vi "chart_combined.vi"() -> ()   [LabVIEW 8.6]
uses:
  Controls/lxw_chart_type.ctl
  Controls/lxw_chart_axis_type.ctl
panel:
  out "error out":errorcluster
  out "function return 2":string
  # "chart_combined.xlsx"
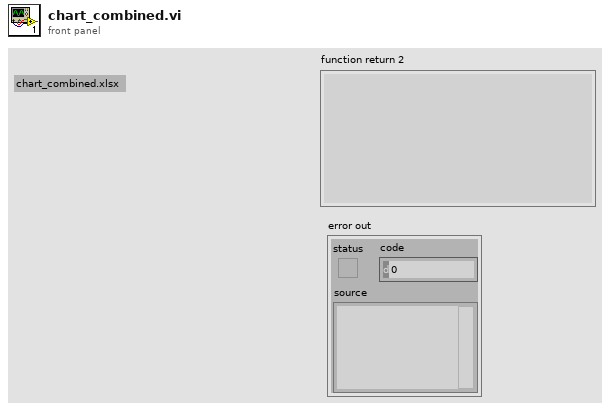
[diagram p1: front panel]
types:
  T1 = typedef "lxw_chart_axis_type.ctl" = u8
  T2 = typedef "lxw_chart_type.ctl" = u8
  T3 = enum32{"invalid app kind", "Development System", "Run Time System", "Student Edition", "Embedded LabVIEW", "Evaluation", "Custom"}
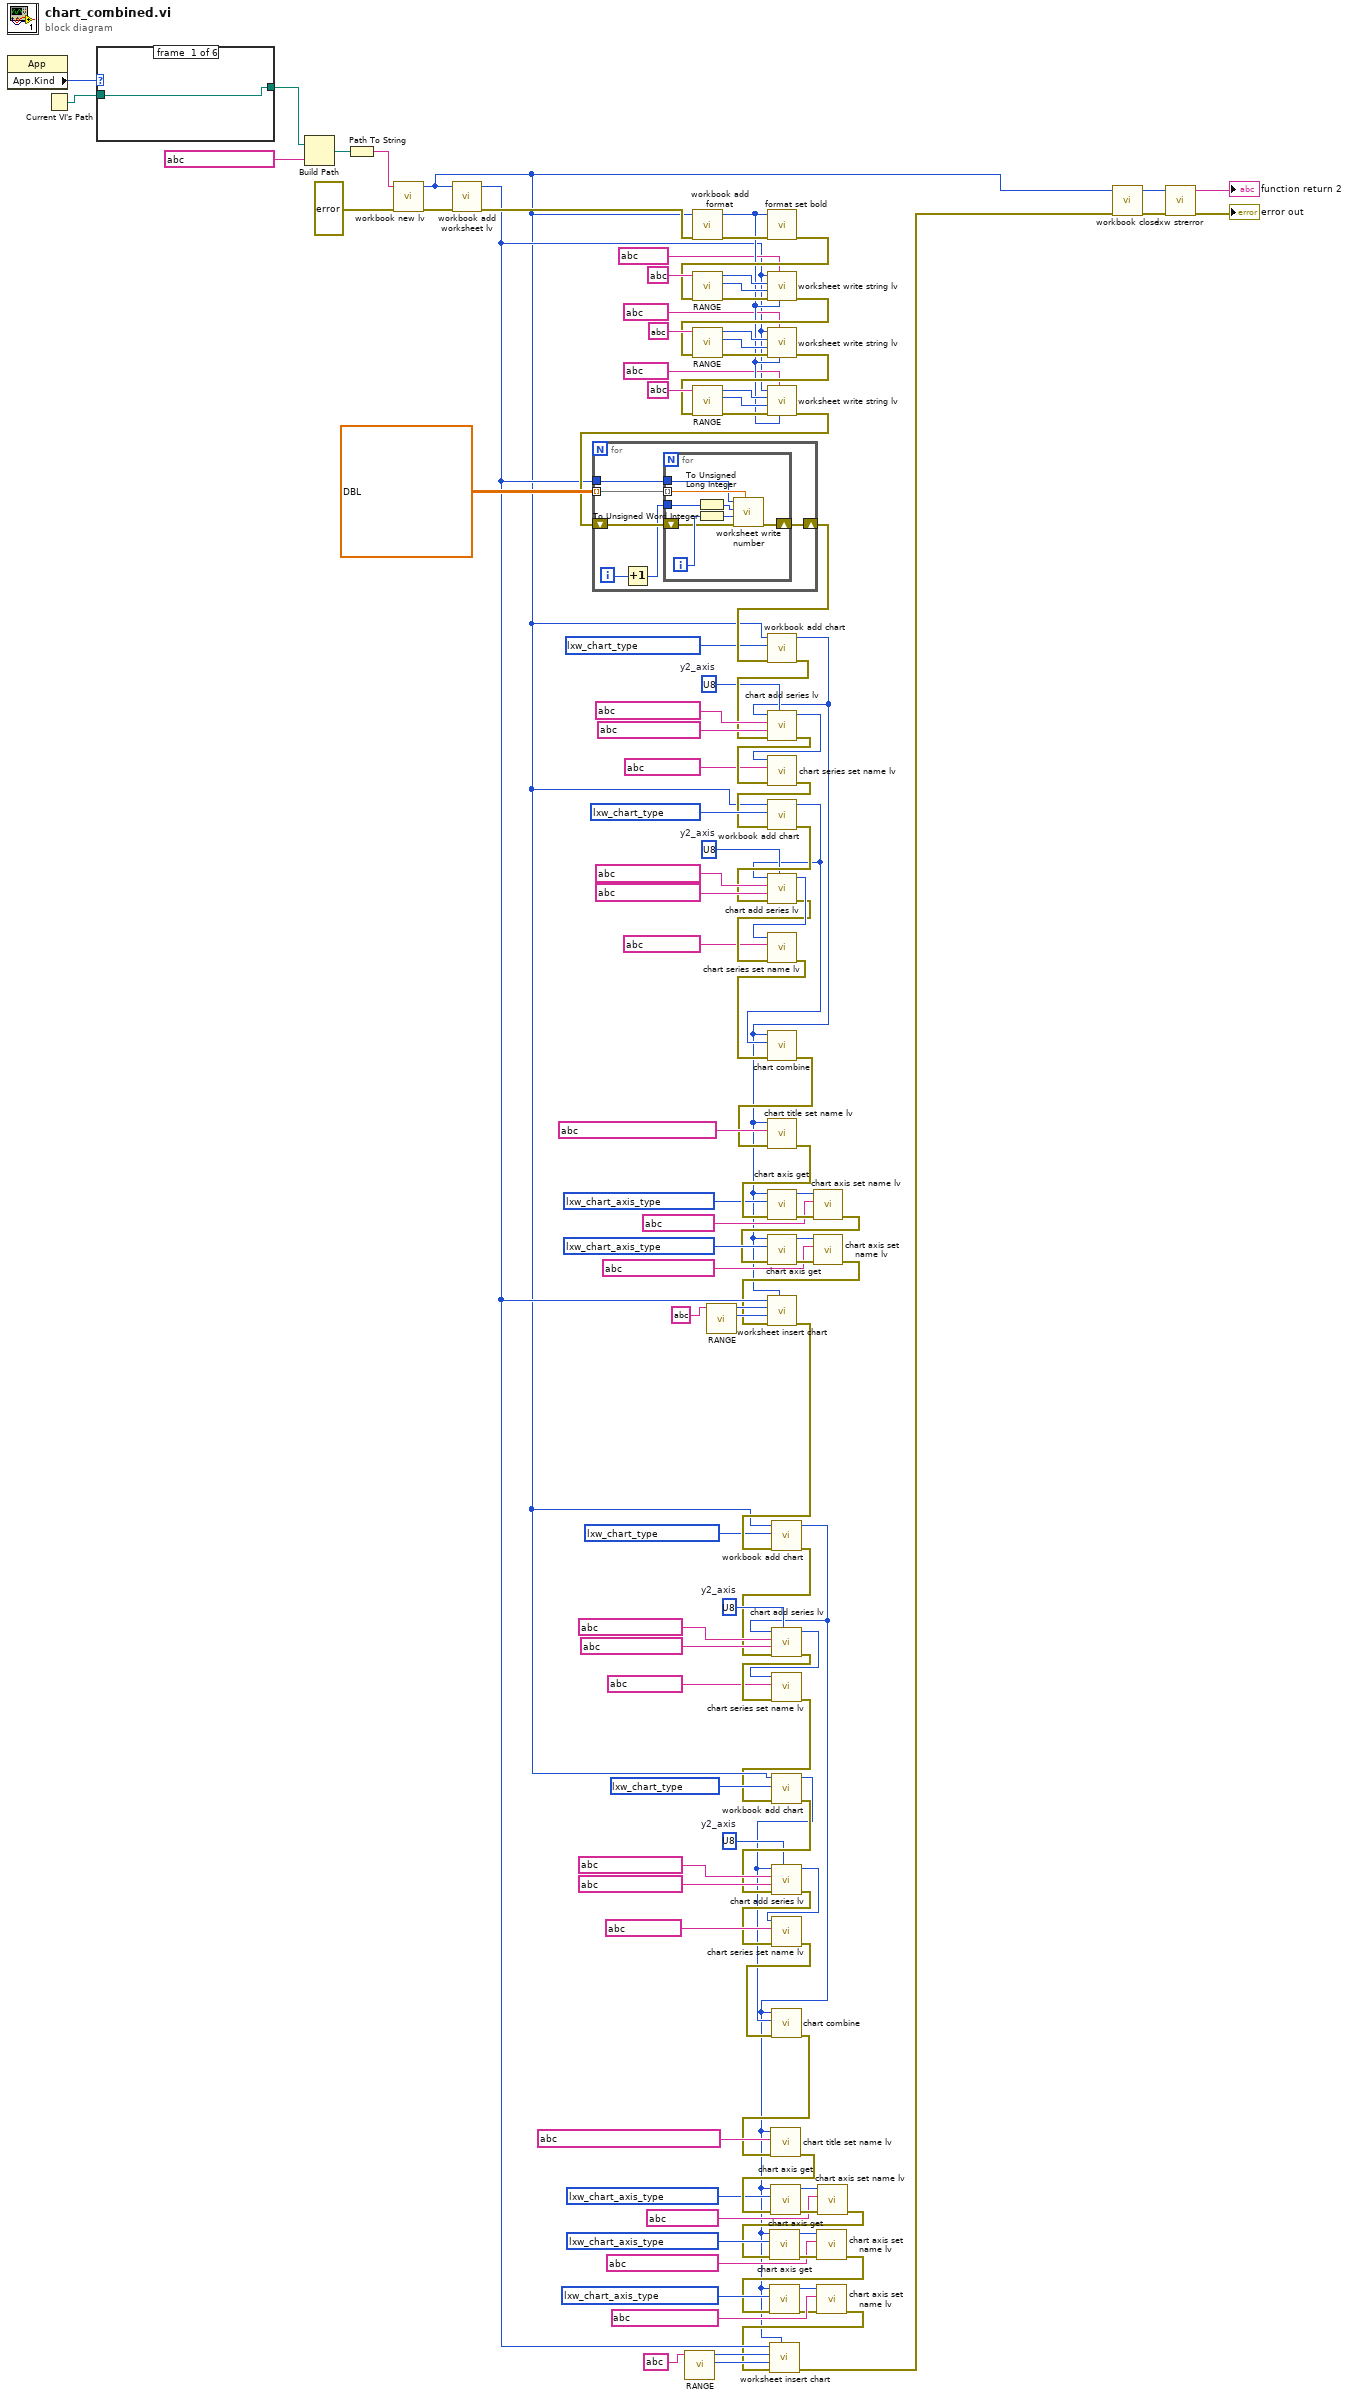
[diagram p0: block diagram]
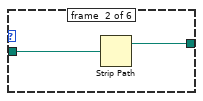
[diagram p2: hidden frame]
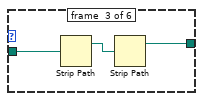
[diagram p3: hidden frame]
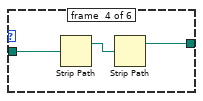
[diagram p4: hidden frame]
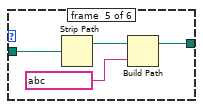
[diagram p5: hidden frame]
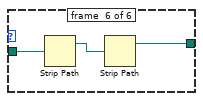
[diagram p6: hidden frame]
diagram:
  w7 = T1 ? items=["LXW_CHART_AXIS_TYPE_X", "LXW_CHART_AXIS_TYPE_Y", "LXW_CHART_AXIS_TYPE_X2", "LXW_CHART_AXIS_TYPE_Y2"] ("axis_type")
  w9 = u8 ?  # y2_axis
  w14 = T2 ? items=["LXW_CHART_NONE", "LXW_CHART_AREA", "LXW_CHART_AREA_STACKED", "LXW_CHART_AREA_STACKED_PERCENT", "LXW_CHART_BAR", "LXW_CHART_BAR_STACKED", "LXW_CHART_BAR_STACKED_PERCENT", "LXW_CHART_COLUMN", "LXW_CHART_COLUMN_STACKED", "LXW_CHART_COLUMN_STACKED_PERCENT", "LXW_CHART_DOUGHNUT", "LXW_CHART_LINE", "LXW_CHART_LINE_STACKED", "LXW_CHART_LINE_STACKED_PERCENT", "LXW_CHART_PIE", "LXW_CHART_SCATTER", "LXW_CHART_SCATTER_STRAIGHT", "LXW_CHART_SCATTER_STRAIGHT_WITH_MARKERS", "LXW_CHART_SCATTER_SMOOTH", "LXW_CHART_SCATTER_SMOOTH_WITH_MARKERS", "LXW_CHART_RADAR", "LXW_CHART_RADAR_WITH_MARKERS", "LXW_CHART_RADAR_FILLED", "LXW_CHART_STOCK"] ("chart_type")
  w21 = T1 ? items=["LXW_CHART_AXIS_TYPE_X", "LXW_CHART_AXIS_TYPE_Y", "LXW_CHART_AXIS_TYPE_X2", "LXW_CHART_AXIS_TYPE_Y2"] ("axis_type")
  w26 = T1 ? items=["LXW_CHART_AXIS_TYPE_X", "LXW_CHART_AXIS_TYPE_Y", "LXW_CHART_AXIS_TYPE_X2", "LXW_CHART_AXIS_TYPE_Y2"] ("axis_type")
  w37 = u8 ?  # y2_axis
  w41 = T2 ? items=["LXW_CHART_NONE", "LXW_CHART_AREA", "LXW_CHART_AREA_STACKED", "LXW_CHART_AREA_STACKED_PERCENT", "LXW_CHART_BAR", "LXW_CHART_BAR_STACKED", "LXW_CHART_BAR_STACKED_PERCENT", "LXW_CHART_COLUMN", "LXW_CHART_COLUMN_STACKED", "LXW_CHART_COLUMN_STACKED_PERCENT", "LXW_CHART_DOUGHNUT", "LXW_CHART_LINE", "LXW_CHART_LINE_STACKED", "LXW_CHART_LINE_STACKED_PERCENT", "LXW_CHART_PIE", "LXW_CHART_SCATTER", "LXW_CHART_SCATTER_STRAIGHT", "LXW_CHART_SCATTER_STRAIGHT_WITH_MARKERS", "LXW_CHART_SCATTER_SMOOTH", "LXW_CHART_SCATTER_SMOOTH_WITH_MARKERS", "LXW_CHART_RADAR", "LXW_CHART_RADAR_WITH_MARKERS", "LXW_CHART_RADAR_FILLED", "LXW_CHART_STOCK"] ("chart_type")
  w49 = u8 ?  # y2_axis
  w52 = T2 ? items=["LXW_CHART_NONE", "LXW_CHART_AREA", "LXW_CHART_AREA_STACKED", "LXW_CHART_AREA_STACKED_PERCENT", "LXW_CHART_BAR", "LXW_CHART_BAR_STACKED", "LXW_CHART_BAR_STACKED_PERCENT", "LXW_CHART_COLUMN", "LXW_CHART_COLUMN_STACKED", "LXW_CHART_COLUMN_STACKED_PERCENT", "LXW_CHART_DOUGHNUT", "LXW_CHART_LINE", "LXW_CHART_LINE_STACKED", "LXW_CHART_LINE_STACKED_PERCENT", "LXW_CHART_PIE", "LXW_CHART_SCATTER", "LXW_CHART_SCATTER_STRAIGHT", "LXW_CHART_SCATTER_STRAIGHT_WITH_MARKERS", "LXW_CHART_SCATTER_SMOOTH", "LXW_CHART_SCATTER_SMOOTH_WITH_MARKERS", "LXW_CHART_RADAR", "LXW_CHART_RADAR_WITH_MARKERS", "LXW_CHART_RADAR_FILLED", "LXW_CHART_STOCK"] ("chart_type")
  w65 = T1 ? items=["LXW_CHART_AXIS_TYPE_X", "LXW_CHART_AXIS_TYPE_Y", "LXW_CHART_AXIS_TYPE_X2", "LXW_CHART_AXIS_TYPE_Y2"] ("axis_type")
  w70 = T1 ? items=["LXW_CHART_AXIS_TYPE_X", "LXW_CHART_AXIS_TYPE_Y", "LXW_CHART_AXIS_TYPE_X2", "LXW_CHART_AXIS_TYPE_Y2"] ("axis_type")
  w74 = u8 ?  # y2_axis
  w80 = T2 ? items=["LXW_CHART_NONE", "LXW_CHART_AREA", "LXW_CHART_AREA_STACKED", "LXW_CHART_AREA_STACKED_PERCENT", "LXW_CHART_BAR", "LXW_CHART_BAR_STACKED", "LXW_CHART_BAR_STACKED_PERCENT", "LXW_CHART_COLUMN", "LXW_CHART_COLUMN_STACKED", "LXW_CHART_COLUMN_STACKED_PERCENT", "LXW_CHART_DOUGHNUT", "LXW_CHART_LINE", "LXW_CHART_LINE_STACKED", "LXW_CHART_LINE_STACKED_PERCENT", "LXW_CHART_PIE", "LXW_CHART_SCATTER", "LXW_CHART_SCATTER_STRAIGHT", "LXW_CHART_SCATTER_STRAIGHT_WITH_MARKERS", "LXW_CHART_SCATTER_SMOOTH", "LXW_CHART_SCATTER_SMOOTH_WITH_MARKERS", "LXW_CHART_RADAR", "LXW_CHART_RADAR_WITH_MARKERS", "LXW_CHART_RADAR_FILLED", "LXW_CHART_STOCK"] ("chart_type")
  n1 = property class="App"() -> ("App.Kind"=w117:T3)  [unwired: 2 in, 2 out]
  n2 = Current VI's Path() -> (path=w116:path)
  n3 = case shown="\"Evaluation\"" w117 {
    tunnel: w116 -> [w118 w120 w123 w126 w130 w133]
    tunnel: [w118 w119 w121 w124 w128 w131] -> w115
    frame #0 {
    }
    frame #1 {
      n4 = Strip Path(path=w120) -> (stripped path=w119:path)  [unwired: 1 out]
    }
    frame #2 {
      n5 = Strip Path(path=w123) -> (stripped path=w122:path)  [unwired: 1 out]
      n6 = Strip Path(path=w122) -> (stripped path=w121:path)  [unwired: 1 out]
    }
    frame #3 {
      n7 = Strip Path(path=w126) -> (stripped path=w125:path)  [unwired: 1 out]
      n8 = Strip Path(path=w125) -> (stripped path=w124:path)  [unwired: 1 out]
    }
    frame #4 {
      n9 = Strip Path(path=w130) -> (stripped path=w129:path)  [unwired: 1 out]
      n10 = Build Path(base path=w129, name or relative path=string ?) -> (appended path=w128:path)
    }
    frame #5 {
      n11 = Strip Path(path=w133) -> (stripped path=w132:path)  [unwired: 1 out]
      n12 = Strip Path(path=w132) -> (stripped path=w131:path)  [unwired: 1 out]
    }
  }
  n13 = Build Path(base path=w115, name or relative path=string ? ("filename")) -> (appended path=w107:path)
  n14 = Path To String(path=w107) -> (string=w106:string)
  n15 = call "workbook new lv.vi"("error in (no error)"=errorcluster ?, "filename"=w106) -> ("error out"=w113:errorcluster, "function return"=w43:u32)  [unwired: 8 in]
  n16 = call "workbook add worksheet lv.vi"("error in (no error)"=w113, "workbook"=w43) -> ("error out"=w85:errorcluster, "function return"=w58:u32)  [unwired: 8 in]
  n17 = call "RANGE.vi"("range_str"=string ?) -> ("col"=w17:u16, "row"=w16:u32)  [unwired: 6 in, 3 out]
  n18 = call "workbook add format.vi"("error in (no error)"=w85, "workbook"=w43) -> ("error out"=w90:errorcluster, "function return"=w88:u32)  [unwired: 8 in]
  n19 = call "RANGE.vi"("range_str"=string ?) -> ("col"=w63:u16, "row"=w62:u32)  [unwired: 6 in, 3 out]
  n20 = call "format set bold.vi"("error in (no error)"=w90, "format"=w88) -> ("error out"=w89:errorcluster)  [unwired: 9 in]
  n21 = call "RANGE.vi"("error in (no error)"=w89, "range_str"=string ?) -> ("error out"=w101:errorcluster, "col"=w97:u16, "row"=w98:u32)  [unwired: 5 in, 2 out]
  n22 = call "worksheet write string lv.vi"("format"=w88, "string"=string ?, "error in (no error)"=w101, "col"=w97, "row"=w98, "worksheet"=w58) -> ("error out"=w92:errorcluster)  [unwired: 4 in, 1 out]
  n23 = call "RANGE.vi"("error in (no error)"=w92, "range_str"=string ?) -> ("error out"=w100:errorcluster, "col"=w95:u16, "row"=w96:u32)  [unwired: 5 in, 2 out]
  n24 = call "worksheet write string lv.vi"("format"=w88, "string"=string ?, "error in (no error)"=w100, "col"=w95, "row"=w96, "worksheet"=w58) -> ("error out"=w91:errorcluster)  [unwired: 4 in, 1 out]
  n25 = call "RANGE.vi"("error in (no error)"=w91, "range_str"=string ?) -> ("error out"=w99:errorcluster, "col"=w93:u16, "row"=w94:u32)  [unwired: 5 in, 2 out]
  n26 = call "worksheet write string lv.vi"("format"=w88, "string"=string ?, "error in (no error)"=w99, "col"=w93, "row"=w94, "worksheet"=w58) -> ("error out"=w86:errorcluster)  [unwired: 4 in, 1 out]
  n27 = for {
    tunnel: dbl[][] ? -> [w139] mode=indexing
    shift-right: [w137] -> w87
    shift-left: w86 -> [w138]
    tunnel: w58 -> [w136]
    i -> [w135]
    n28 = Increment(x=w135) -> (x+1=w134:i32)
    n29 = for {
      tunnel: w139 -> [w147] mode=indexing
      tunnel: w134 -> [w144]
      shift-right: [w141] -> w137
      shift-left: w138 -> [w142]
      tunnel: w136 -> [w140]
      i -> [w146]
      n30 = To Unsigned Long Integer(number=w144) -> (unsigned 32bit integer=w143:u32)
      n31 = To Unsigned Word Integer(number=w146) -> (unsigned 16bit integer=w145:u16)
      n32 = call "worksheet write number.vi"("number"=w147, "error in (no error)"=w142, "col"=w145, "row"=w143, "worksheet"=w140) -> ("error out"=w141:errorcluster)  [unwired: 5 in, 1 out]
    }
  }
  n33 = call "workbook add chart.vi"("error in (no error)"=w87, "chart_type"=w80, "workbook"=w43) -> ("error out"=w75:errorcluster, "function return"=w42:u32)  [unwired: 7 in]
  n34 = call "chart add series lv.vi"("y2_axis"=w74, "error in (no error)"=w75, "values"=string ?, "categories"=string ?, "chart"=w42) -> ("error out"=w79:errorcluster, "function return"=w73:u32)  [unwired: 5 in]
  n35 = call "chart series set name lv.vi"("error in (no error)"=w79, "name"=string ? ("values"), "series"=w73) -> ("error out"=w51:errorcluster)  [unwired: 8 in]
  n36 = call "workbook add chart.vi"("error in (no error)"=w51, "chart_type"=w52, "workbook"=w43) -> ("error out"=w50:errorcluster, "function return"=w48:u32)  [unwired: 7 in]
  n37 = call "chart add series lv.vi"("y2_axis"=w49, "error in (no error)"=w50, "values"=string ? ("range_str"), "categories"=string ? ("range_str"), "chart"=w48) -> ("error out"=w56:errorcluster, "function return"=w57:u32)  [unwired: 5 in]
  n38 = call "chart series set name lv.vi"("error in (no error)"=w56, "name"=string ? ("range_str"), "series"=w57) -> ("error out"=w47:errorcluster)  [unwired: 8 in]
  n39 = call "chart combine.vi"("error in (no error)"=w47, "combined_chart"=w48, "chart"=w42) -> ("error out"=w46:errorcluster)  [unwired: 8 in]
  n40 = call "chart title set name lv.vi"("error in (no error)"=w46, "name"=string ?, "chart"=w42) -> ("error out"=w71:errorcluster)  [unwired: 8 in]
  n41 = call "chart axis get.vi"("error in (no error)"=w71, "axis_type"=w70, "chart"=w42) -> ("error out"=w68:errorcluster, "function return"=w69:u32)  [unwired: 7 in]
  n42 = call "chart axis set name lv.vi"("error in (no error)"=w68, "name"=string ?, "axis"=w69) -> ("error out"=w64:errorcluster)  [unwired: 8 in]
  n43 = call "chart axis get.vi"("error in (no error)"=w64, "axis_type"=w65, "chart"=w42) -> ("error out"=w67:errorcluster, "function return"=w66:u32)  [unwired: 7 in]
  n44 = call "chart axis set name lv.vi"("error in (no error)"=w67, "name"=string ?, "axis"=w66) -> ("error out"=w45:errorcluster)  [unwired: 8 in]
  n45 = call "worksheet insert chart.vi"("chart"=w42, "error in (no error)"=w45, "col"=w63, "row"=w62, "worksheet"=w58) -> ("error out"=w81:errorcluster)  [unwired: 5 in, 1 out]
  n46 = call "workbook add chart.vi"("error in (no error)"=w81, "chart_type"=w41, "workbook"=w43) -> ("error out"=w35:errorcluster, "function return"=w2:u32)  [unwired: 7 in]
  n47 = call "chart add series lv.vi"("y2_axis"=w37, "error in (no error)"=w35, "values"=string ?, "categories"=string ?, "chart"=w2) -> ("error out"=w40:errorcluster, "function return"=w30:u32)  [unwired: 5 in]
  n48 = call "chart series set name lv.vi"("error in (no error)"=w40, "name"=string ? ("values"), "series"=w30) -> ("error out"=w13:errorcluster)  [unwired: 8 in]
  n49 = call "workbook add chart.vi"("error in (no error)"=w13, "chart_type"=w14, "workbook"=w43) -> ("error out"=w12:errorcluster, "function return"=w3:u32)  [unwired: 7 in]
  n50 = call "chart add series lv.vi"("y2_axis"=w9, "error in (no error)"=w12, "values"=string ?, "categories"=string ?, "chart"=w3) -> ("error out"=w31:errorcluster, "function return"=w29:u32)  [unwired: 5 in]
  n51 = call "chart series set name lv.vi"("error in (no error)"=w31, "name"=string ? ("values"), "series"=w29) -> ("error out"=w11:errorcluster)  [unwired: 8 in]
  n52 = call "chart combine.vi"("error in (no error)"=w11, "combined_chart"=w3, "chart"=w2) -> ("error out"=w10:errorcluster)  [unwired: 8 in]
  n53 = call "chart title set name lv.vi"("error in (no error)"=w10, "name"=string ?, "chart"=w2) -> ("error out"=w27:errorcluster)  [unwired: 8 in]
  n54 = call "chart axis get.vi"("error in (no error)"=w27, "axis_type"=w26, "chart"=w2) -> ("error out"=w24:errorcluster, "function return"=w25:u32)  [unwired: 7 in]
  n55 = call "chart axis set name lv.vi"("error in (no error)"=w24, "name"=string ?, "axis"=w25) -> ("error out"=w20:errorcluster)  [unwired: 8 in]
  n56 = call "chart axis get.vi"("error in (no error)"=w20, "axis_type"=w21, "chart"=w2) -> ("error out"=w23:errorcluster, "function return"=w22:u32)  [unwired: 7 in]
  n57 = call "chart axis set name lv.vi"("error in (no error)"=w23, "name"=string ?, "axis"=w22) -> ("error out"=w5:errorcluster)  [unwired: 8 in]
  n58 = call "chart axis get.vi"("error in (no error)"=w5, "axis_type"=w7, "chart"=w2) -> ("error out"=w6:errorcluster, "function return"=w1:u32)  [unwired: 7 in]
  n59 = call "chart axis set name lv.vi"("error in (no error)"=w6, "name"=string ?, "axis"=w1) -> ("error out"=w4:errorcluster)  [unwired: 8 in]
  n60 = call "worksheet insert chart.vi"("chart"=w2, "error in (no error)"=w4, "col"=w17, "row"=w16, "worksheet"=w58) -> ("error out"=w44:errorcluster)  [unwired: 5 in, 1 out]
  n61 = call "workbook close.vi"("error in (no error)"=w44, "workbook"=w43) -> ("error out"=w109:errorcluster, "function return"=w111:u32)  [unwired: 8 in]
  n62 = call "lxw strerror.vi"("error in (no error)"=w109, "error_num"=w111) -> ("error out"=→"error out":errorcluster, "function return"=→"function return 2":string)  [unwired: 8 in]
